vi "niRFUtil RFHS Channelizer ReadBuffer CSG.vi"(0 "Buffer":csg[](array[numeric]), 5 "Index":i32, 7 "Length":i32) -> (6 "Data":csg[](array[numeric]))   [LabVIEW 2015, in "niRFUtil.lvlib"]
uses:
  niRFUtil.lvlib
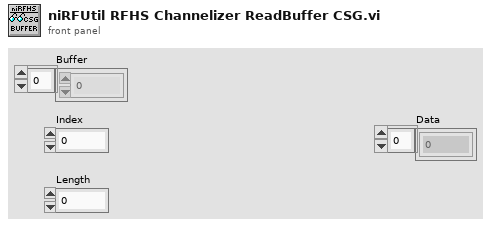
[diagram p1: front panel]
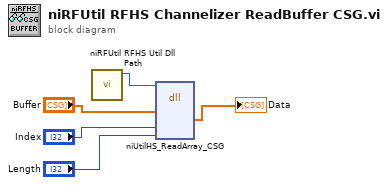
[diagram p0: block diagram]
diagram:
  n1 = call "niRFUtil RFHS Util Dll Path.vi"() -> ("Path"=w1:path)  [unwired: 7 in, 4 out]
  n2 = dll-call lib="?" fn="niUtilHS_ReadArray_CSG"(path in=w1, "buf"="Buffer", "index"="Index", "length"="Length") -> ("Data"=→"Data":csg[])  [unwired: 7 in, 2 out]
